vi "Get File Rename Paths.vi"(8 "error in":errorcluster, 9 "plugin file extension":string, 10 "plugin name":string, 11 "plugin library path":path) -> (0 "error out":errorcluster, 2 "new file path":path, 3 "old file path":path)   [LabVIEW 2021, in "InstrumentStudio Plug-In Editor.lvlib"]
uses:
  InstrumentStudio Plug-In Editor.lvlib
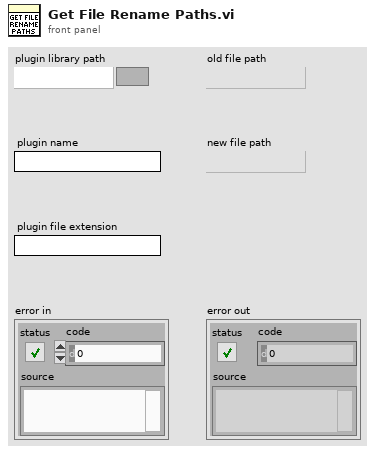
[diagram p1: front panel]
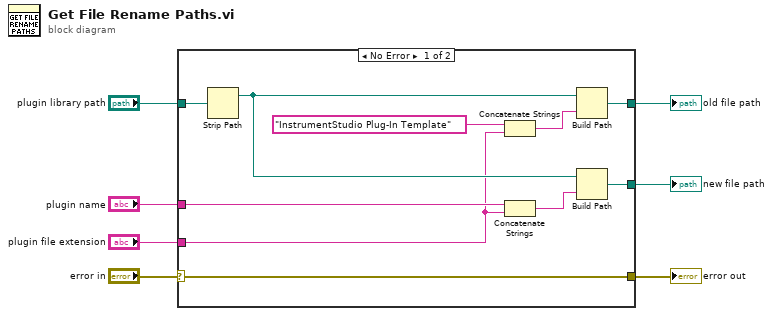
[diagram p0: block diagram]
diagram:
  n1 = case shown="No Error" "error in" {
    selector: "error in" -> [w8 w18]
    tunnel: "plugin name" -> [w16 _]
    tunnel: [w12 _] -> w6
    tunnel: "plugin file extension" -> [w11 _]
    tunnel: [w10 _] -> w4
    tunnel: "plugin library path" -> [w9 _]
    tunnel: [w8 w18] -> w2
    frame No Error {
      n2 = Strip Path(path=w9) -> (stripped path=w13:path)  [unwired: 1 out]
      n3 = Concatenate Strings("InstrumentStudio Plug-In Template" ("string"), w11) -> (w14:string)
      n4 = Concatenate Strings(w16, w11) -> (w15:string)
      n5 = Build Path(base path=w13, name or relative path=w14) -> (appended path=w12:path)
      n6 = Build Path(base path=w13, name or relative path=w15) -> (appended path=w10:path)
    }
    frame Error {
    }
  }
  "new file path" <- w4
  "old file path" <- w6
  "error out" <- w2
